vi "New Table From Document.vi"(7 "xwpfTable in":refnum<class "xwpfTable.lvclass">, 8 "error in (no error)":errorcluster, 11 "Table Ref":refnum<k24>) -> (0 "error out":errorcluster, 3 "xwpfTable out":refnum<class "xwpfTable.lvclass">)   [LabVIEW 2017, in "Word_Specific.lvlib" / "xwpfTable.lvclass"]
uses:
  xwpfTable.lvclass
  C:/Users/Neo/Desktop/Dev_Tools_BR/LabVIEW_NPOI/lib/NPOI 2.1.1/NPOI.OOXML.dll
  lib/NPOI 2.1.1/NPOI.OOXML.dll
  xwpfTable.lvclass/xwpfTable.ctl
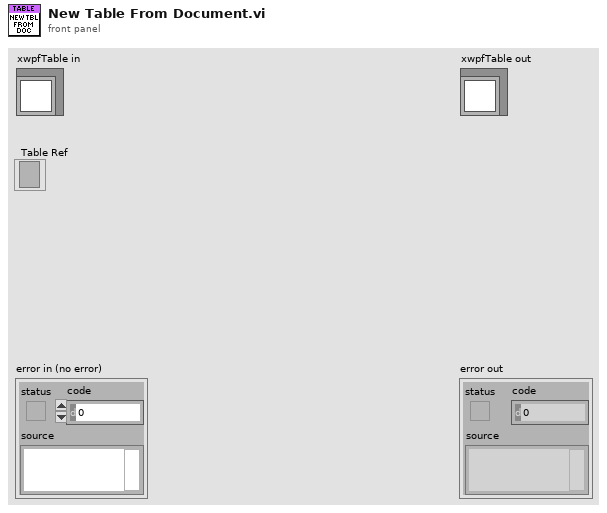
[diagram p1: front panel]
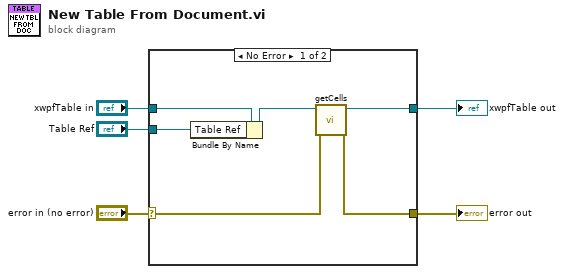
[diagram p0: block diagram]
diagram:
  n1 = case shown="No Error" "error in (no error)" {
    selector: "error in (no error)" -> [w7 w13]
    tunnel: [w6 w13] -> w4
    tunnel: [w8 w12] -> w2
    tunnel: "xwpfTable in" -> [w11 w12]
    tunnel: "Table Ref" -> [w10 _]
    frame No Error {
      n2 = Bundle By Name(cluster=w11, "Table Ref"=w10) -> (w9:refnum<class "xwpfTable.lvclass">)
      n3 = call "getCells.vi"("error in (no error)"=w7, "xwpfTable in"=w9) -> ("error out"=w6:errorcluster, "xwpfTable out"=w8:refnum<class "xwpfTable.lvclass">)  [unwired: 8 in]
    }
    frame Error {
    }
  }
  "error out" <- w4
  "xwpfTable out" <- w2
